vi "Protocole_envoie_bruit_2020.vi"() -> ()   [LabVIEW 2020]
uses:
  bfbeb452-2a3a-4e65-bf29-1a1bdd43f38b.vi
  fdb60019-a1c3-41cd-bca7-4044fe2d6920.vi
  <vilib>/numeric/Random Number (Range) DBL.vi
  0129e9be-af5f-4d34-b4ce-d6aa148f68f5.vi
  20c94d61-f86f-453d-a01a-8f3ee0d40214.vi
  0a7551a9-e03c-499c-be3b-b63e1f9fbd9c.vi
  <vilib>/Analysis/1siggen.llb/General Gauss-Mod Sine.vi
  <vilib>/measure/NI_MABase.lvlib
  <vilib>/Analysis/NI_AALBase.lvlib
panel:
  in  "Control temps bruit à 0":cluster{"Fs":dbl, "#s":dbl}={"Fs"=1000.0, "#s"=1000.0} {"Fs" format="%.2p"}
  in  "Control temps bruit":cluster{"Fs":dbl, "#s":dbl}={"Fs"=1000.0, "#s"=1000.0} {"Fs" format="%.2p"}
  in  "Control temps son à 0":cluster{"Fs":dbl, "#s":dbl}={"Fs"=1000.0, "#s"=1000.0} {"Fs" format="%.2p"}
  in  "Nom du fichier":string="Test_"
  out "Barre de progression":dbl(slide) scale=0.0..100.0
  in  "?":enum32{"Temps", "Numérique "}(tab)
  in  "Temps d'attente entre chaque sons /s":dbl=2.0
  in  "Plus ou moins /s":dbl=1.0
  in  "Nombre de répétition d'opération":dbl=1.0
  in  "Nombre de sons":dbl=3.0
  in  "Amplitude min /V":dbl=0.5
  in  "Différence entre chaque amplitude /V":dbl=0.2
  in  "Lieu du fichier":path=path "D:/Labview/Stage/LabVIEW 2020/Programmes_utilisables/Protocoles_enregistrement_ampli/Protocole_envoie_bruit_2020/Donnees" caption="Filename"
  in  "Control temps son":cluster{"Fs":dbl, "#s":dbl}={"Fs"=1000.0, "#s"=1000.0} {"Fs" format="%.2p"}
  in  "?":bool=TRUE
  in  "?":bool
  in  "?":enum32{"Sons", "Bruit"}(tab)
  in  "Fréquence /Hz":dbl=440.0
  in  "Type de son":u64(knob) scale=0.0..3.0
  in  "Temps du son /s":dbl=0.5
  in  "Temps du bruit /s":dbl=0.1
  # "Bruit"
  # "Sons"
  # "Protocole :"
  # "Pas touché"
  # "Triangle"
  # "Carré"
  # "Dents de scie"
  # "Sinus"
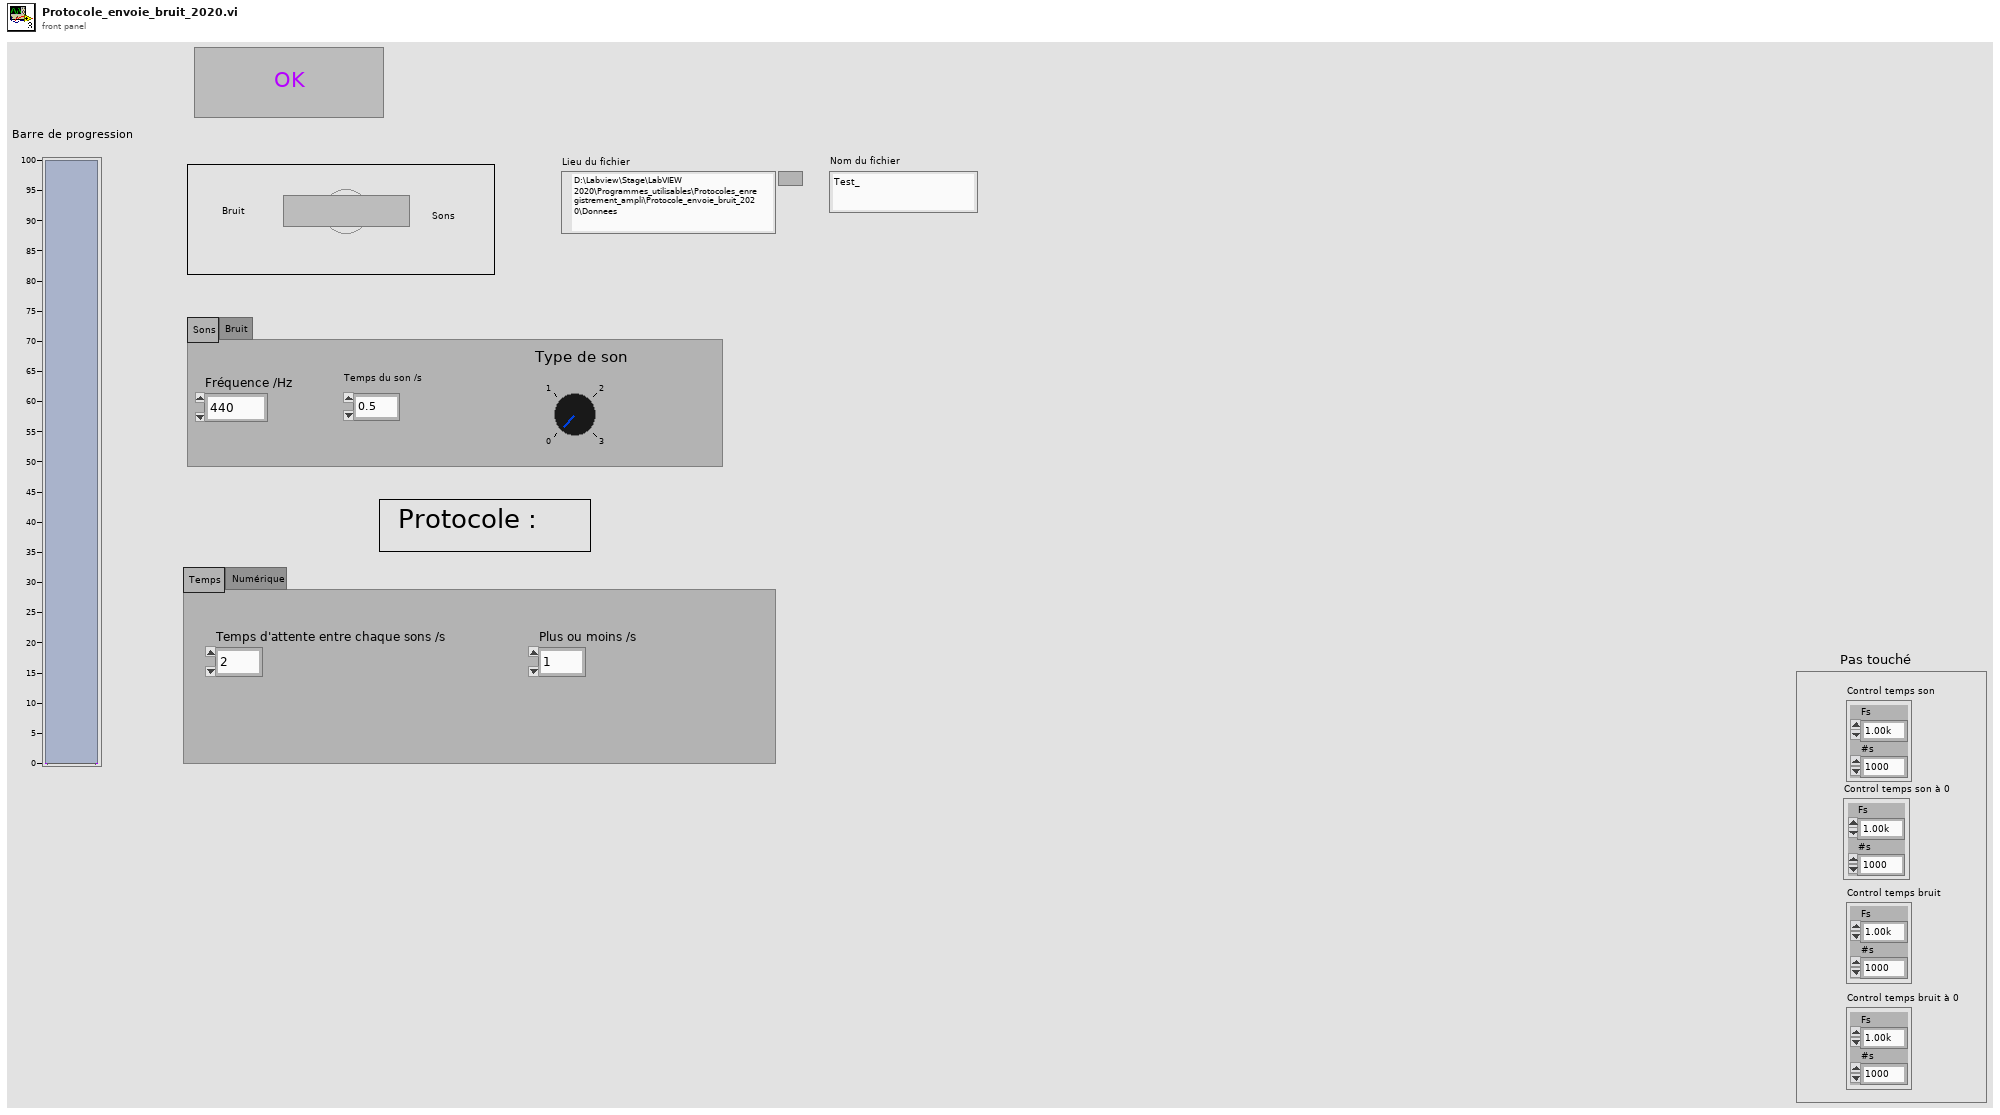
[diagram p1: front panel]
types:
  T1 = enum16{"open", "open or create", "create or replace", "create", "open (read-only)"}
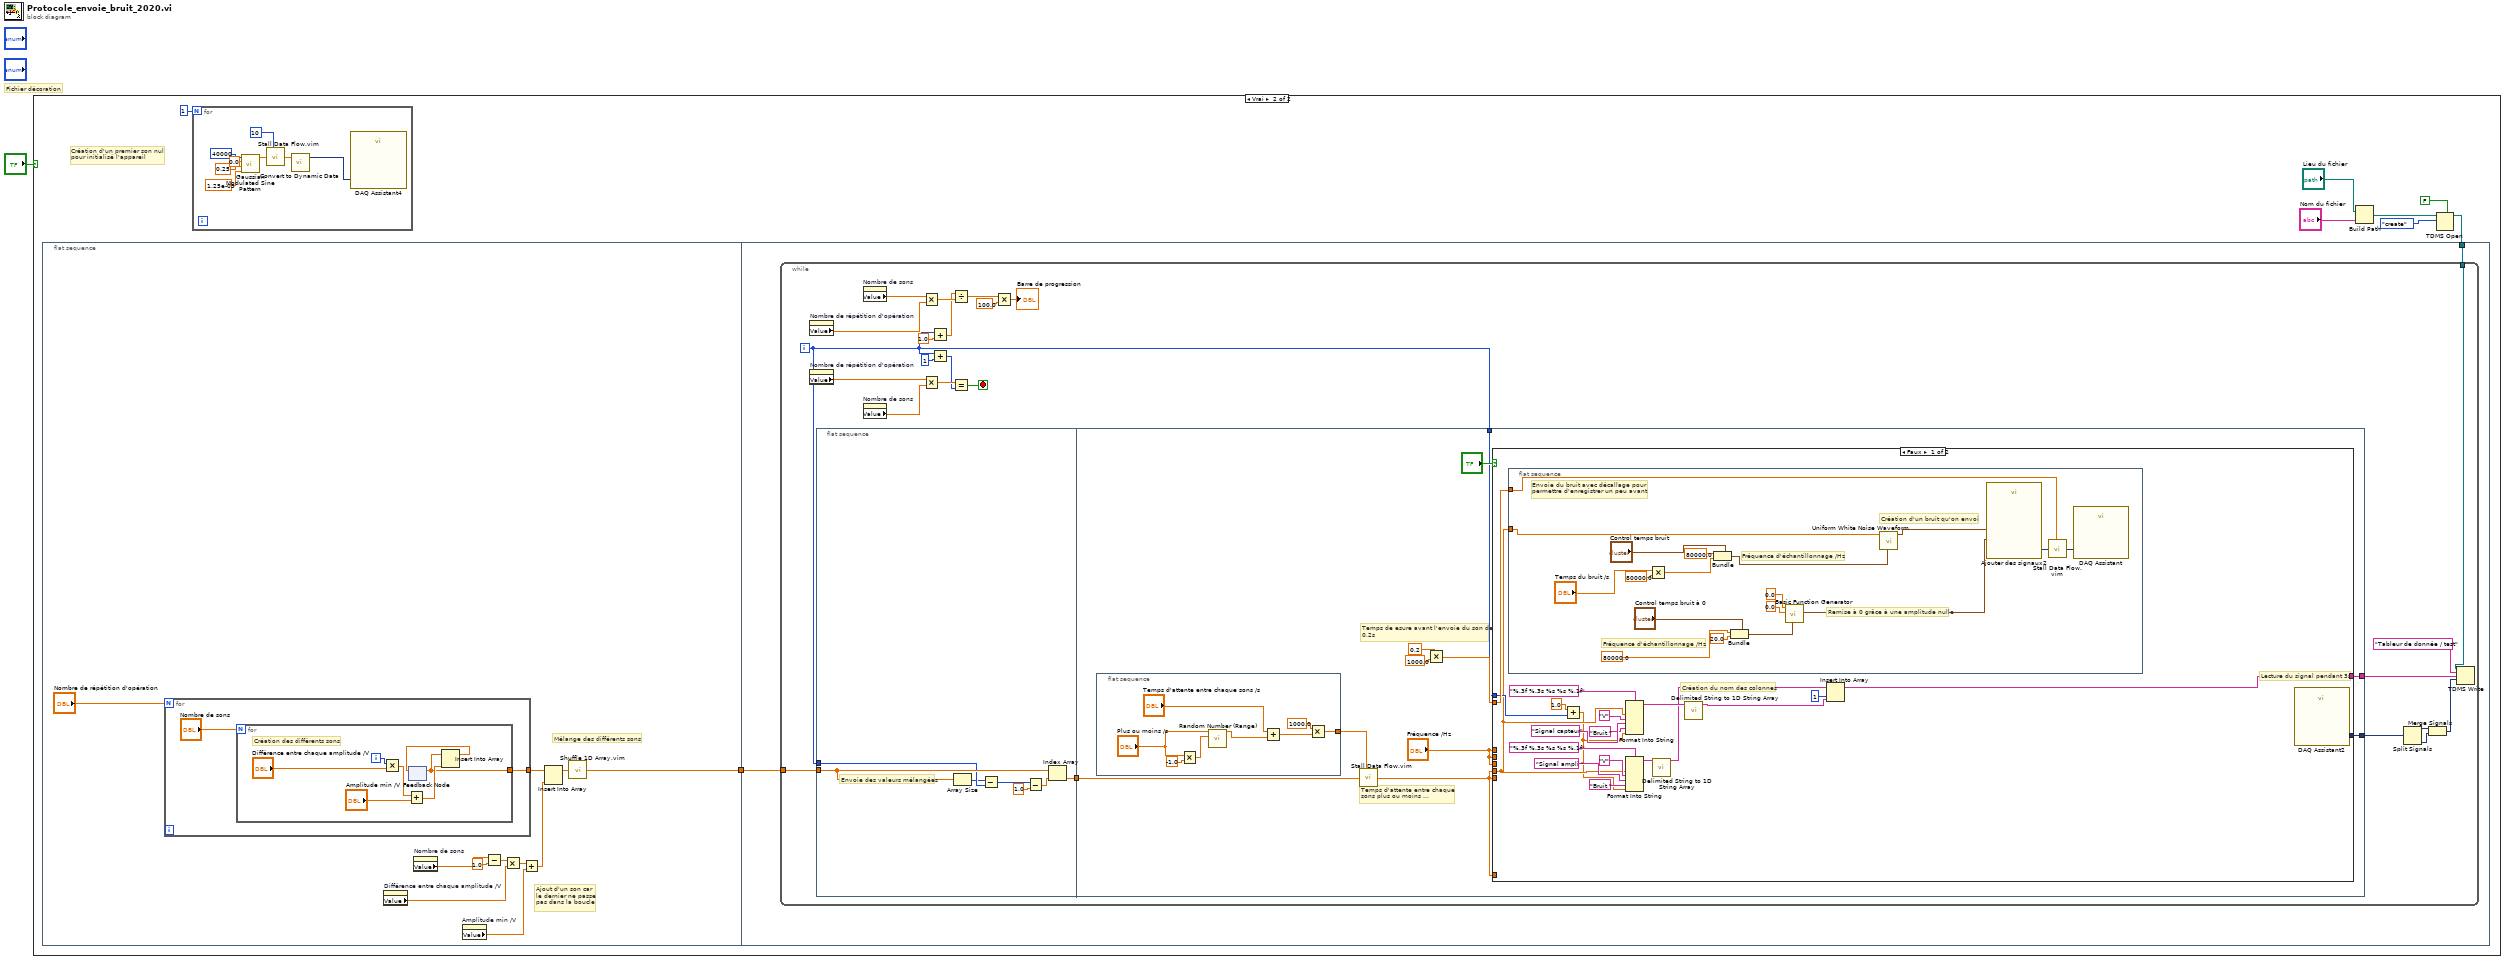
[diagram p0: block diagram]
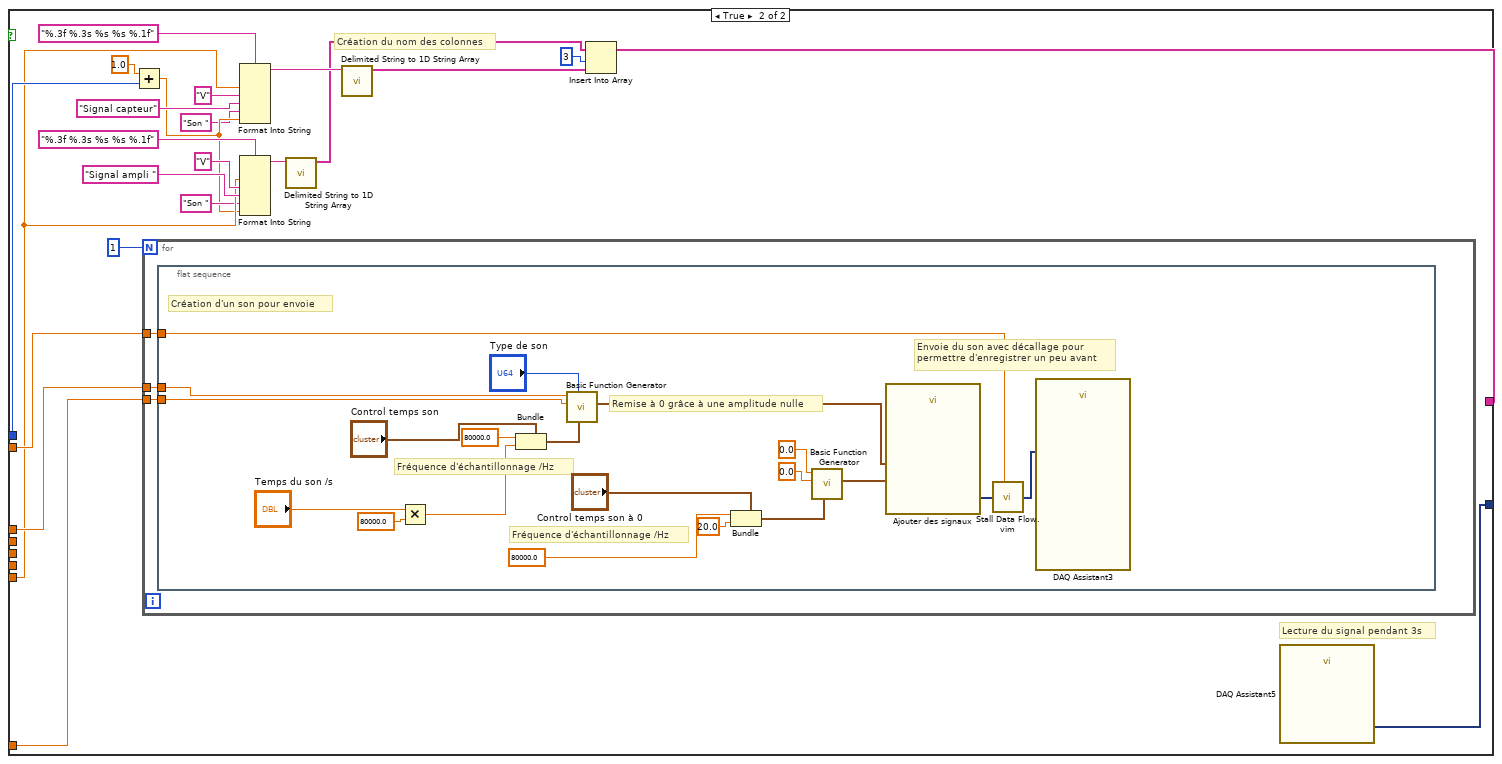
[diagram p3: hidden frame]
diagram:
  # "Fichier décoration"
  n1 = case shown="Vrai" "?" {
    frame False {
    }
    frame True {
      # "Création d'un premier son nul\npour initialisé l'appareil"
      n2 = flat-sequence {
        tunnel: [w19] -> w9
        tunnel: w9 -> [w39]
        tunnel: w8 -> [w38]
        frame #0 {
          # "Mélange des différents sons"
          # "Ajout d'un son car \nle dernier ne passe \npas dans la boucle"
          n3 = for {
            N: "Nombre de répétition d'opération" -> [_]
            tunnel: [w29] -> w18
            n4 = for {
              N: "Nombre de sons" -> [_]
              tunnel: [w32] -> w29
              i -> [w36]
              # "Création des différents sons"
              n5 = Multiply(x=w36, y="Différence entre chaque amplitude /V") -> (x*y=w37:dbl)
              n6 = Add(x=w37, y="Amplitude min /V") -> (x+y=w33:dbl)
              n7 = feedback #1() -> (w32:dbl[])  [unwired: 1 in]
              n8 = Insert Into Array(array=w32, new element=w33) -> (w31:dbl[])  [unwired: 1 in]
              n9 = feedback-in #1(w31) -> ()
            }
          }
          n10 = property on="Différence entre chaque amplitude /V" class="NumNb (strict)"() -> ("Value"=w25:dbl)  [unwired: 2 in, 2 out]
          n11 = property on="Nombre de sons" class="NumNb (strict)"() -> ("Value"=w22:dbl)  [unwired: 2 in, 2 out]
          n12 = property on="Amplitude min /V" class="NumNb (strict)"() -> ("Value"=w23:dbl)  [unwired: 2 in, 2 out]
          n13 = Subtract(x=w22, y=1.0) -> (x-y=w20:dbl)
          n14 = Multiply(x=w20, y=w25) -> (x*y=w24:dbl)
          n15 = Add(x=w24, y=w23) -> (x+y=w27:dbl)
          n16 = Insert Into Array(array=w18, new element=w27) -> (w26:dbl[])  [unwired: 1 in]
          n17 = call "Shuffle 1D Array.vim"("array"=w26) -> ("shuffled array"=w19:dbl[])  [unwired: 4 in]
        }
        frame #1 {
          n18 = while {
            tunnel: w39 -> [w44]
            tunnel: w38 -> [w49]
            i -> [w46]
            stop <- w60 stop-if-true
            n19 = property on="Nombre de répétition d'opération" class="NumNb (strict)"() -> ("Value"=w56:dbl)  [unwired: 2 in, 2 out]
            n20 = property on="Nombre de répétition d'opération" class="NumNb (strict)"() -> ("Value"=w63:dbl)  [unwired: 2 in, 2 out]
            n21 = flat-sequence {
              tunnel: w44 -> [w70]
              tunnel: w46 -> [w69]
              tunnel: [w67] -> w59
              tunnel: w59 -> [w73]
              tunnel: [w76] -> w43
              tunnel: [w75] -> w47
              tunnel: w46 -> [w74]
              frame #0 {
                # "Envoie des valeurs mélangées"
                n22 = Array Size(array=w70) -> (size(s)=w68:i32)
                n23 = Subtract(x=w68, y=w69) -> (x-y=w65:i32)
                n24 = Subtract(x=w65, y=1.0) -> (x-y=w64:dbl)
                n25 = Index Array(array=w70, index=w64) -> (element=w67:dbl)
              }
              frame #1 {
                # "Temps de esure avant l'envoie du son de \n0,2s"
                # "Temps d'attente entre chaque \nsons plus ou moins ..."
                n26 = flat-sequence {
                  tunnel: [w85] -> w72
                  frame #0 {
                    n27 = Multiply(x="Plus ou moins /s", y=-1.0) -> (x*y=w84:dbl)
                    n28 = call-poly <vilib>:"Random Number (Range).vi"("lower bound (0)"=w84, "upper bound (100)"="Plus ou moins /s") -> ("number"=w82:dbl)  [unwired: 9 in]
                    n29 = Add(x="Temps d'attente entre chaque sons /s", y=w82) -> (x+y=w89:dbl)
                    n30 = Multiply(x=1000.0, y=w89) -> (x*y=w85:dbl)
                  }
                }
                n31 = call "Stall Data Flow.vim"("value in"=w73, "milliseconds to wait"=w72) -> ("value out"=w77:dbl)  [unwired: 1 out]
                n32 = Multiply(x=0.2, y=1000.0) -> (x*y=w80:dbl)
                n33 = case shown="Faux" "?" {
                  tunnel: "Fréquence /Hz" -> [_ w150]
                  tunnel: w77 -> [_ w149]
                  tunnel: w77 -> [w93 _]
                  tunnel: w80 -> [w109 w148]
                  tunnel: "Fréquence /Hz" -> [_ _]
                  tunnel: w77 -> [_ w135]
                  tunnel: "Fréquence /Hz" -> [_ _]
                  tunnel: [w108 w142] -> w76
                  tunnel: [w96 w132] -> w75
                  tunnel: w74 -> [w95 w140]
                  frame False {
                    # "Création du nom des colonnes"
                    # "Lecture du signal pendant 3s"
                    n34 = flat-sequence {
                      tunnel: w93 -> [w112]
                      tunnel: w109 -> [w121]
                      frame #0 {
                        # "Remise à 0 grâce à une amplitude nulle"
                        # "Création d'un bruit qu'on envoi"
                        # "Fréquence d'échantillonnage /Hz"
                        # "Envoie du bruit avec décallage pour \npermettre d'enregistrer un peu avant"
                        # "Fréquence d'échantillonnage /Hz"
                        n35 = Multiply(x="Temps du bruit /s", y=80000.0) -> (x*y=w125:dbl)
                        n36 = Bundle(cluster="Control temps bruit", "Fs"=80000.0, "#s"=w125) -> (w111:cluster{"Fs":dbl, "#s":dbl})
                        n37 = Bundle(cluster="Control temps bruit à 0", "Fs"=80000.0, "#s"=20.0) -> (w115:cluster{"Fs":dbl, "#s":dbl})
                        n38 = call <vilib>:"Basic Function Generator.vi"("sampling info"=w115, "amplitude"=0.0, "frequency"=0.0) -> ("signal out"=w120:waveform(dbl))  [unwired: 6 in, 2 out]
                        n39 = call <vilib>:"Uniform White Noise Waveform.vi"("sampling info"=w111, "amplitude"=w112) -> ("signal out"=w110:waveform(dbl))  [unwired: 8 in, 1 out]
                        n40 = call "Ajouter des signaux2"("Input Signal B"=w120, "Input Signal A"=w110) -> ("Appended Signals"=w113:dynamicdata)  [unwired: 8 in, 1 out]
                        n41 = call "Stall Data Flow.vim"("value in"=w113, "milliseconds to wait"=w121) -> ("value out"=w122:dynamicdata)  [unwired: 1 out]
                        n42 = call "DAQ Assistant"("data"=w122) -> ()  [unwired: 17 in, 2 out]
                      }
                    }
                    n43 = Add(x=1.0, y=w95) -> (x+y=w91:dbl)
                    n44 = Format Into String(format string="%.3f %.3s %s %s %.1f" ("chaîne de format"), w93, "V" ("entrée 2"), "Signal capteur" ("entrée 2"), "Bruit " ("entrée 4"), w91) -> (resulting string=w105:string)  [unwired: 2 in, 1 out]
                    n45 = Format Into String(format string="%.3f %.3s %s %s %.1f" ("chaîne de format"), w93, "V" ("entrée 2"), "Signal ampli " ("entrée 2"), "Bruit " ("entrée 4"), w91) -> (resulting string=w107:string)  [unwired: 2 in, 1 out]
                    n46 = call <vilib>:"Delimited String to 1D String Array.vi"("delimited string"=w107) -> ("string array"=w94:string[])  [unwired: 10 in]
                    n47 = call <vilib>:"Delimited String to 1D String Array.vi"("delimited string"=w105) -> ("string array"=w98:string[])  [unwired: 10 in]
                    n48 = Insert Into Array(array=w94, index=1, new element=w98) -> (w96:string[])
                    n49 = call "DAQ Assistant2"() -> ("data"=w108:dynamicdata)  [unwired: 17 in, 2 out]
                  }
                  frame True {
                    # "Création du nom des colonnes"
                    # "Lecture du signal pendant 3s"
                    n50 = Add(x=1.0, y=w140) -> (x+y=w129:dbl)
                    n51 = for {
                      N: 1 -> [_]
                      tunnel: w150 -> [w151]
                      tunnel: w149 -> [w152]
                      tunnel: w148 -> [w153]
                      n52 = flat-sequence {
                        tunnel: w153 -> [w167]
                        tunnel: w152 -> [w164]
                        tunnel: w151 -> [w163]
                        frame #0 {
                          # "Remise à 0 grâce à une amplitude nulle"
                          # "Création d'un son pour envoie"
                          # "Fréquence d'échantillonnage /Hz"
                          # "Envoie du son avec décallage pour \npermettre d'enregistrer un peu avant"
                          # "Fréquence d'échantillonnage /Hz"
                          n53 = Multiply(x="Temps du son /s", y=80000.0) -> (x*y=w170:dbl)
                          n54 = Bundle(cluster="Control temps son", "Fs"=80000.0, "#s"=w170) -> (w171:cluster{"Fs":dbl, "#s":dbl})
                          n55 = call <vilib>:"Basic Function Generator.vi"("sampling info"=w171, "signal type"="Type de son", "amplitude"=w164, "frequency"=w163) -> ("signal out"=w154:waveform(dbl))  [unwired: 5 in, 2 out]
                          n56 = Bundle(cluster="Control temps son à 0", "Fs"=80000.0, "#s"=20.0) -> (w159:cluster{"Fs":dbl, "#s":dbl})
                          n57 = call <vilib>:"Basic Function Generator.vi"("sampling info"=w159, "amplitude"=0.0, "frequency"=0.0) -> ("signal out"=w156:waveform(dbl))  [unwired: 6 in, 2 out]
                          n58 = call "Ajouter des signaux"("Input Signal B"=w156, "Input Signal A"=w154) -> ("Appended Signals"=w157:dynamicdata)  [unwired: 8 in, 1 out]
                          n59 = call "Stall Data Flow.vim"("value in"=w157, "milliseconds to wait"=w167) -> ("value out"=w173:dynamicdata)  [unwired: 1 out]
                          n60 = call "DAQ Assistant3"("data"=w173) -> ()  [unwired: 17 in, 2 out]
                        }
                      }
                    }
                    n61 = Format Into String(format string="%.3f %.3s %s %s %.1f" ("chaîne de format"), w135, "V" ("entrée 2"), "Signal capteur" ("entrée 2"), "Son " ("entrée 4"), w129) -> (resulting string=w144:string)  [unwired: 2 in, 1 out]
                    n62 = Format Into String(format string="%.3f %.3s %s %s %.1f" ("chaîne de format"), w135, "V" ("entrée 2"), "Signal ampli " ("entrée 2"), "Son " ("entrée 4"), w129) -> (resulting string=w146:string)  [unwired: 2 in, 1 out]
                    n63 = call <vilib>:"Delimited String to 1D String Array.vi"("delimited string"=w146) -> ("string array"=w131:string[])  [unwired: 10 in]
                    n64 = call <vilib>:"Delimited String to 1D String Array.vi"("delimited string"=w144) -> ("string array"=w134:string[])  [unwired: 10 in]
                    n65 = Insert Into Array(array=w131, index=3, new element=w134) -> (w132:string[])
                    n66 = call "DAQ Assistant5"() -> ("data"=w142:dynamicdata)  [unwired: 17 in, 2 out]
                  }
                }
              }
            }
            n67 = property on="Nombre de sons" class="NumNb (strict)"() -> ("Value"=w55:dbl)  [unwired: 2 in, 2 out]
            n68 = property on="Nombre de sons" class="NumNb (strict)"() -> ("Value"=w62:dbl)  [unwired: 2 in, 2 out]
            n69 = Multiply(x=w55, y=w56) -> (x*y=w54:dbl)
            n70 = Multiply(x=w63, y=w62) -> (x*y=w61:dbl)
            n71 = Add(x=w46, y=1.0) -> (x+y=w50:dbl)
            n72 = Add(x=w46, y=1) -> (x+y=w57:i32)
            n73 = Divide(x=w50, y=w54) -> (x/y=w52:dbl)
            n74 = Equal?(x=w61, y=w57) -> (x = y?=w60:bool)
            n75 = Multiply(x=w52, y=100.0) -> (x*y=→"Barre de progression":dbl)
            n76 = Split Signals(w43) -> (w42:dynamicdata, w41:dynamicdata)  [unwired: 4 in, 2 out]
            n77 = Merge Signals(w42, w41) -> (w40:dynamicdata)
            n78 = TDMS Write(0:w49, 5:"Tableur de donnée / test" ("nom du groupe en entrée (Sans titre)"), 7:w47, 9:w40) -> ()  [unwired: 2 in, 4 out]
          }
        }
      }
      n79 = for {
        N: 1 -> [_]
        n80 = call <vilib>:"Gaussian Modulated Sine Pattern.vi"("delta t (s)"=1.25e-05, "delay (s)"=0.25, "amplitude"=0.0, "samples"=40000) -> ("Gauss-Mod Sine Pattern"=w17:dbl[])  [unwired: 6 in, 1 out]
        n81 = call "Stall Data Flow.vim"("value in"=w17, "milliseconds to wait"=u32 10) -> ("value out"=w16:dbl[])  [unwired: 1 out]
        n82 = call "Convert to Dynamic Data"("Array"=w16) -> ("Dynamic Data Type"=w10:dynamicdata)  [unwired: 3 in]
        n83 = call "DAQ Assistant4"("data"=w10) -> ()  [unwired: 17 in, 2 out]
      }
      n84 = Build Path(base path="Lieu du fichier", name or relative path="Nom du fichier") -> (appended path=w5:path)
      n85 = TDMS Open(5:FALSE ("créer un fichier index ? (V)"), 10:T1."create" ("opération (0 : open)"), 11:w5) -> (3:w8:refnum<k34>)  [unwired: 4 in, 1 out]
    }
  }
